vi "CRYResonance Lev-Mar xx.vi"(0 "X":dbl[](array[numeric]) format="%.2f", 1 "Y":dbl[](array[numeric]) format="%.2f", 2 "Coefficients":dbl[](array[numeric]) format="%.2f", 3 "error":i32, 4 "Standard Deviation":dbl[](array[numeric]) format="%.2f") -> (5 "chiSqr":dbl format="%.2f")   [LabVIEW 2013]
panel:
  # "Lev-Mar\nXX"
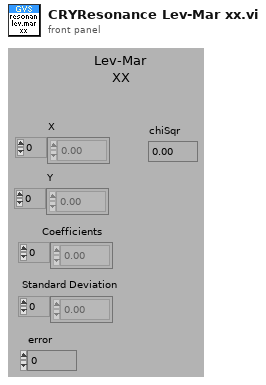
[diagram p1: front panel]
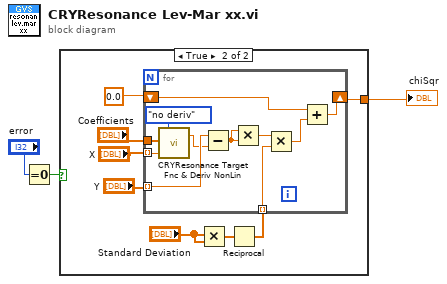
[diagram p0: block diagram]
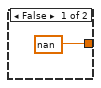
[diagram p2: hidden frame]
diagram:
  n1 = Equal To 0?(x="error") -> (x = 0?=w2:bool)
  n2 = case shown="True" w2 {
    tunnel: [nan w11] -> w1
    frame False {
    }
    frame True {
      n3 = Multiply(x="Standard Deviation", y="Standard Deviation") -> (x*y=w6:dbl[])
      n4 = Reciprocal(x=w6) -> (1/x=w5:dbl[])
      n5 = for {
        shift-right: [w22] -> w11
        shift-left: 0.0 -> [w23]
        tunnel: "Y" -> [w21] mode=indexing
        tunnel: "Coefficients" -> [w19]
        tunnel: "X" -> [w18] mode=indexing
        tunnel: w5 -> [w13] mode=indexing
        n6 = call "CRYResonance Target Fnc & Deriv NonLin.vi"("X"=w18, "Coefficients"=w19, "Flag"=enum16{"no deriv", "deriv"}."no deriv") -> ("Y"=w17:dbl)  [unwired: 1 out]
        n7 = Subtract(x=w21, y=w17) -> (x-y=w20:dbl)
        n8 = Multiply(x=w20, y=w20) -> (x*y=w14:dbl)
        n9 = Multiply(x=w14, y=w13) -> (x*y=w15:dbl)
        n10 = Add(x=w23, y=w15) -> (x+y=w22:dbl)
      }
    }
  }
  "chiSqr" <- w1
